vi "Database-DeleteTypeSelector.vi"(0 "General Instruction":bool, 1 "SQL Statement":string, 2 "error in (no error)":errorcluster, 5 "Manufacturing-Part Number":string) -> (6 "SQL":string, 7 "error out":errorcluster)   [LabVIEW 2013, in "PartCertDatabase-Actor.lvclass"]
uses:
  PartCertDatabase-Actor.lvclass
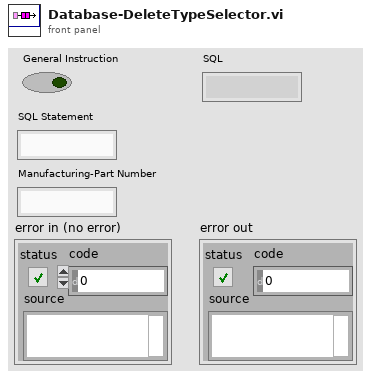
[diagram p1: front panel]
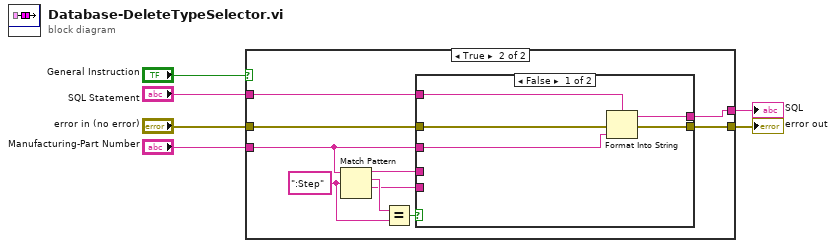
[diagram p0: block diagram]
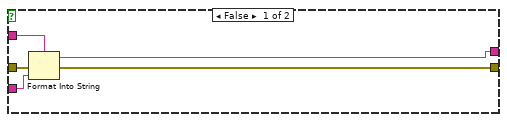
[diagram p2: hidden frame]
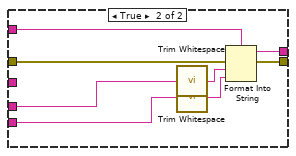
[diagram p3: hidden frame]
diagram:
  n1 = case shown="True" "General Instruction" {
    tunnel: [w11 w18] -> w1
    tunnel: "Manufacturing-Part Number" -> [w10 w12]
    tunnel: "SQL Statement" -> [w9 w21]
    tunnel: "error in (no error)" -> [w8 w20]
    tunnel: [w7 w19] -> w5
    frame False {
      n2 = Format Into String(format string=w9, error in=w8, w10) -> (resulting string=w11:string, error out=w7:errorcluster)  [unwired: 1 in]
    }
    frame True {
      w15 = ":Step" ("regular expression")
      n3 = Match Pattern(string=w12, regular expression=w15) -> (before substring=w14:string, match substring=w16:string, after substring=w13:string)  [unwired: 1 in, 1 out]
      n4 = Equal?(x=w16, y=w15) -> (x = y?=w17:bool)
      n5 = case shown="False" w17 {
        tunnel: w21 -> [w26 w34]
        tunnel: w20 -> [w25 w31]
        tunnel: [w24 w30] -> w19
        tunnel: [w23 w29] -> w18
        tunnel: w14 -> [_ w28]
        tunnel: w13 -> [_ w27]
        tunnel: w12 -> [w22 _]
        frame False {
          n6 = Format Into String(format string=w26, error in=w25, w22) -> (resulting string=w23:string, error out=w24:errorcluster)  [unwired: 1 in]
        }
        frame True {
          n7 = call <vilib>:"Trim Whitespace.vi"("string"=w28) -> ("trimmed string"=w33:string)  [unwired: 1 in]
          n8 = call <vilib>:"Trim Whitespace.vi"("string"=w27) -> ("trimmed string"=w32:string)  [unwired: 1 in]
          n9 = Format Into String(format string=w34, error in=w31, w33, w32) -> (resulting string=w29:string, error out=w30:errorcluster)  [unwired: 1 in]
        }
      }
    }
  }
  "error out" <- w5
  "SQL" <- w1
